vi "PH_Beckhoff_PP_Control.write Mercury to PSDB.vi"(0 "i ref in":refnum<vi>, 5 "error IO":errorcluster) -> (14 "i ref out":refnum<vi>, 19 "error out":errorcluster)   [LabVIEW 2014, in "PH_Beckhoff_PP_Control.lvlib"]
doc: "This VI writes the mercury data to the PHELIX shot data base."
uses:
  PH_Beckhoff_PP_Control.lvlib
  PH_Basics/PH_StatusHandler/PH_StatusHandler.Status.ctl
  PH_Basics/PH_PSDBWriter/PH_PSDBWriter.Data Status.ctl
  PH_Beckhoff/PH_Beckhoff.lvlib
  CS_Core/CSSystem/CSSystemLib/CSSystemLib.lvlib
  PH_Basics/PH_PSDBWriter/PH_PSDBWriter.lvlib
  PH_Basics/PH_Common/PH_Common.lvlib
  PH_Basics/PH_StatusHandler/PH_StatusHandler.lvlib
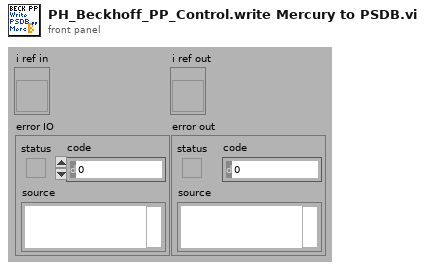
[diagram p1: front panel]
types:
  T1 = typedef "PH_Beckhoff.lvlib/PH_Beckhoff.i attribute.ctl" = cluster{"GUI Refs":T2, "operation?":bool, "Default Prdc Interval":i32, "Connection":T3, "AMS Net ID":T4, "Klemmencluster: # of":T5, "Values":T6, "IP":string, "Description":string, "configured?":bool, "Change Manager":cluster{"Detemination wanted?":bool, "Values changed at":cluster{"Sonderklemmen Inputs":i32[], "Analog Inputs":i32[], "Analog Outputs":i32[], "Digital Inputs":i32[], "Digital Outputs":i32[]}}, "Difference to handle an analog input as change":u32}
  T2 = typedef "PH_Beckhoff.lvlib/PH_Beckhoff.GUI Refs.ctl" = cluster{"ADS Error":refnum<vi>, "Values":refnum<vi>, "configured?":refnum<vi>, "Connection":refnum<vi>, "IP":refnum<vi>, "Prdc Int [ms]":refnum<vi>}
  T3 = typedef "PH_Beckhoff.lvlib/PH_Beckhoff.Connectivity.ctl" = cluster{"DLL?":bool, "Port?":bool, "Client?":bool, "Ping?":bool, "unsuccessful Pings":u32}
  T4 = typedef "Beckhoff - Driver np.lvlib/Beckhoff Access.ctl" = cluster{"DLL path":path, "AMS Net ID":cluster{"1st # of IP":u8, "2nd # of IP":u8, "3rd # of IP":u8, "4th # of IP":u8, "In Port":u8, "Out Port":u8}}
  T5 = typedef "Beckhoff - Driver np.lvlib/Klemmendeclarer.ctl" = cluster{"Offset due to Sonderklemms":u32, "analog Inputs":u32, "analog Outputs":u32, "digital Input Bits":u32, "digital Output Bits":u32}
  T6 = typedef "PH_Beckhoff.lvlib/PH_Beckhoff.Values.ctl" = cluster{"Sonderklemmen Inputs":T7, "Analog Inputs":T8, "Analog Outputs":T10, "Digital Inputs":T11, "Digital Outputs":T12}
  T7 = typedef "PH_Beckhoff.lvlib/PH_Beckhoff.Sonderklemmen Inputs.ctl" = cluster{"Total Length":u32, "Name":string, "Value":u64, "Quality":bool, "Service ID":i32, "Offset":u32, "Length":u32}[]
  T8 = typedef "PH_Beckhoff.lvlib/PH_Beckhoff.Analog Inputs.ctl" = cluster{"Name":string, "Value":u32, "Quality":bool, "Service ID":i32, "Sca Type":T9}[]
  T9 = typedef "PH_Beckhoff.lvlib/PH_Beckhoff.Scaling Type.ctl" = enum16{"none", "0 ... 15 Bit -> 0 ... 5", "0 ... 15 Bit -> 0 ... 10", "0 ... 15 Bit -> 0 ... 25", "0 ... 15 Bit -> 4 ... 20", "0 ... 15 Bit -> 0 ... 1", "0 ... 15 Bit -> 0 ... 20000", "0 ... 15 Bit -> 0 ... 24000"}
  T10 = typedef "PH_Beckhoff.lvlib/PH_Beckhoff.Analog Outputs.ctl" = cluster{"Name":string, "Value":u32, "Quality":bool, "Wanted Value":u32, "Service ID":i32, "Sca Type":T9}[]
  T11 = typedef "PH_Beckhoff.lvlib/PH_Beckhoff.Digital Inputs.ctl" = cluster{"Name":string, "Value":bool, "Quality":bool, "Service ID":i32, "inverted?":bool}[]
  T12 = typedef "PH_Beckhoff.lvlib/PH_Beckhoff.Digital Outputs.ctl" = cluster{"Name":string, "Value":bool, "Quality":bool, "Wanted Value":bool, "Service ID":i32, "inverted?":bool}[]
  T13 = typedef "PH_Beckhoff_PP_Control.lvlib/PH_Beckhoff_PP_Control.i attribute.ctl" = cluster{"PP Conductivity Control":cluster{"PSDB":cluster{"Status Service ID":i32, "Instance ID":i32, "Data Status":T14, "Ref Status":refnum<vi>, "Error Code":i32}, "Status":cluster{"GUI Ref":refnum<vi>, "Status Service ID":i32, "Status":T15}, "DIs":cluster{"Device on":cluster{"GUI Ref":refnum<vi>, "# in Data":i32}, "Conductivity ok":cluster{"GUI Ref":refnum<vi>, "# in Data":i32}, "Temperature ok":cluster{"GUI Ref":refnum<vi>, "# in Data":i32}, "Alarm":cluster{"GUI Ref":refnum<vi>, "# in Data":i32}}, "PSDB Thread":cluster{"Ref":refnum<vi>, "Q-Ref":refnum<queue>}}, "PP Mercury Control":cluster{"PSDB":cluster{"Status Service ID":i32, "Instance ID":i32, "Data Status":T14, "Ref Status":refnum<vi>, "Error Code":i32}, "Status":cluster{"GUI Ref":refnum<vi>, "Status Service ID":i32, "Status":T15}, "on since:":cluster{"GUI Ref":refnum<vi>, "Service ID":i32, "Time":string}, "DIs":cluster{"Device on":cluster{"GUI Ref":refnum<vi>, "# in Data":i32}, "Alarm":cluster{"GUI Ref":refnum<vi>, "# in Data":i32}}, "AIs":cluster{"Concentration":cluster{"GUI Ref":refnum<vi>, "# in Data":i32}}, "PSDB Thread":cluster{"Ref":refnum<vi>, "Q-Ref":refnum<queue>}}, "PSDB":cluster{"Shot #":i32, "Subsystem":T16}, "PSDB Credentials":T17}
  T14 = typedef "PH_PSDBWriter.lvlib/PH_PSDBWriter.Data Status.ctl" = i16
  T15 = typedef "PH_StatusHandler.lvlib/PH_StatusHandler.Status.ctl" = i16
  T16 = typedef "PH_PSDBWriter.lvlib/PH_PSDBWriter.PHELIX-Subsystems.ctl" = i32
  T17 = typedef "PH_Common.lvlib/PH_Connection.PSDB Credentials.ctl" = cluster{"PW":string, "ID":string, "DS":string}
  T18 = typedef "PH_PSDBWriter.lvlib/PH_PSDBWriter.Numeric dataset.ctl" = cluster{"name":string, "data":dbl, "unit":string}
  T19 = typedef "PH_PSDBWriter.lvlib/PH_PSDBWriter.String dataset.ctl" = cluster{"name":string, "data":string, "unit":string}
  T20 = typedef "PH_PSDBWriter.lvlib/PH_PSDBWriter.PSDB Dataset.ctl" = cluster{"Version":i32, "2D data Input":T21[], "Boolean Input":T23[], "Image Input":T24[], "Numeric Input":T18[], "String Input":T19[]}
  T21 = typedef "PH_PSDBWriter.lvlib/PH_PSDBWriter.2D dataset.ctl" = cluster{"name":string, "data":dbl[][], "axis description":T22}
  T22 = typedef "PSDB.lvlib/PSDB_AxisDescription.ctl" = cluster{"x axis label":string, "y axis label":string, "x axis unit":string, "y axis unit":string}
  T23 = typedef "PH_PSDBWriter.lvlib/PH_PSDBWriter.Boolean dataset.ctl" = cluster{"name":string, "data":bool, "unit":string}
  T24 = typedef "PH_PSDBWriter.lvlib/PH_PSDBWriter.Image dataset.ctl" = cluster{"name":string, "data":T25, "unit":string}
  T25 = typedef "IMAQ Image.ctl" = refnum<image>
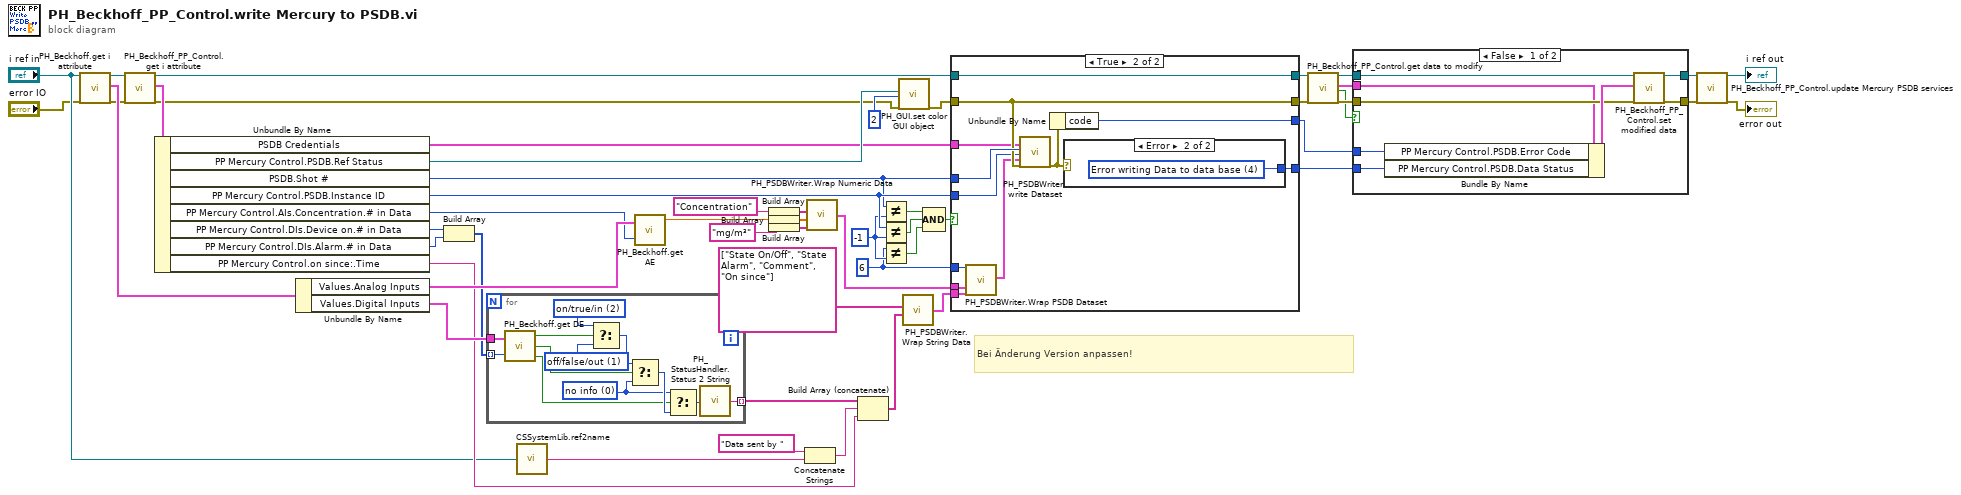
[diagram p0: block diagram]
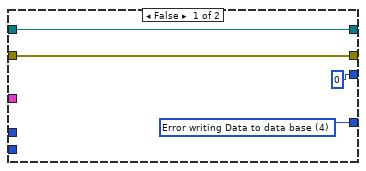
[diagram p3: hidden frame]
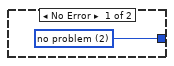
[diagram p4: hidden frame]
diagram:
  w41 = 6 ("Version")
  w47 = -1 ("y")
  # "Bei Änderung Version anpassen!"
  n1 = call "PH_Beckhoff.get i attribute.vi"("i ref in"="i ref in", "error in (no error)"="error IO") -> ("i ref out"=w40:refnum<vi>, "i attribute"=w39:T1, "error out"=w19:errorcluster)  [unwired: 15 in]
  n2 = call "PH_Beckhoff_PP_Control.get i attribute.vi"("i ref in"=w40, "error in (no error)"=w19) -> ("i ref out"=w20:refnum<vi>, "i attribute"=w16:T13, "error out"=w13:errorcluster)  [unwired: 15 in]
  n3 = Unbundle By Name(w16) -> ("PSDB Credentials"=w1:T17, "PP Mercury Control.PSDB.Ref Status"=w14:refnum<vi>, "PSDB.Shot #"=w50:i32, "PP Mercury Control.PSDB.Instance ID"=w51:i32, "PP Mercury Control.AIs.Concentration.# in Data"=w37:i32, "PP Mercury Control.DIs.Device on.# in Data"=w35:i32, "PP Mercury Control.DIs.Alarm.# in Data"=w34:i32, "PP Mercury Control.on since:.Time"=w28:string)
  n4 = Unbundle By Name(w39) -> ("Values.Analog Inputs"=w38:T8, "Values.Digital Inputs"=w36:T11)
  n5 = Build Array(w35, w34) -> (w33:i32[])
  n6 = for {
    tunnel: [w59] -> w32 mode=indexing
    tunnel: w36 -> [w55]
    tunnel: w33 -> [w54] mode=indexing
    w61 = T15 1 items=["no info", "off/false/out", "on/true/in", "Failure", "Alarm", "Status 1", "Status 2", "Status 3"] ("State Temp not 2 low")
    w62 = T15 2 items=["no info", "off/false/out", "on/true/in", "Failure", "Alarm", "Status 1", "Status 2", "Status 3"] ("State Temp not 2 low")
    w64 = T15 0 items=["no info", "off/false/out", "on/true/in", "Failure", "Alarm", "Status 1", "Status 2", "Status 3"] ("State Temp not 2 low")
    n7 = call "PH_Beckhoff.get DE.vi"("Digital Values"=w55, "index of element"=w54) -> ("Value"=w58:bool, "Quality"=w57:bool, "Tag not found"=w56:bool)
    n8 = Select(t=w62, s=w58, f=w61) -> (s? t:f=w63:T15)
    n9 = Select(t=w63, s=w57, f=w64) -> (s? t:f=w65:T15)
    n10 = Select(t=w64, s=w56, f=w65) -> (s? t:f=w60:T15)
    n11 = call "PH_StatusHandler.Status 2 String.vi"("Status"=w60) -> ("Status as string"=w59:string)
  }
  n12 = call "CSSystemLib.ref2name.vi"("obj refnum"="i ref in") -> ("name"=w30:string)
  n13 = call "PH_Beckhoff.get AE.vi"("Analog Inputs"=w38, "index of element"=w37) -> ("DIM value"=w9:dbl)  [unwired: 2 out]
  n14 = Build Array("Concentration" ("name")) -> (w6:string[])
  n15 = Build Array(w9) -> (w8:dbl[])
  n16 = Build Array("mg/m³" ("unit")) -> (w4:string[])
  n17 = Concatenate Strings("Data sent by " ("string"), w30) -> (w29:string)
  n18 = call "PH_PSDBWriter.Wrap Numeric Data.vi"("Unit Array"=w4, "Data Array"=w8, "Name Array"=w6) -> ("PSDB Numeric Data Array"=w3:T18[])  [unwired: 1 in]
  n19 = Build Array (concatenate)(w32, w29, w28) -> (w10:string[])
  n20 = Not Equal?(x=w50, y=w47) -> (x != y?=w46:bool)
  n21 = Not Equal?(x=w51, y=w47) -> (x != y?=w45:bool)
  n22 = Not Equal?(x=w41, y=w47) -> (x != y?=w44:bool)
  n23 = call "PH_GUI.set color GUI object.vi"("GUI object Ref"=w14, "State"=2, "error in (no error)"=w13) -> ("error out"=w12:errorcluster)  [unwired: 16 in]
  n24 = call "PH_PSDBWriter.Wrap String Data.vi"("Data Array"=w10, "Name Array"=string[] ["State On/Off", "State Alarm", "Comment", "On since"]) -> ("PSDB String Data Array"=w2:T19[])  [unwired: 2 in]
  n25 = Compound Arithmetic op=AND(w46, w45, w44) -> (w43:bool)
  n26 = case shown="True" w43 {
    tunnel: w12 -> [w67 w77]
    tunnel: w51 -> [_ w74]
    tunnel: w41 -> [_ w71]
    tunnel: [w69 w81] -> w48
    tunnel: w20 -> [w68 w80]
    tunnel: [w68 w80] -> w26
    tunnel: [w67 w77] -> w24
    tunnel: w50 -> [_ w78]
    tunnel: [0 ("code") w79] -> w42
    tunnel: w3 -> [_ w73]
    tunnel: w2 -> [_ w72]
    tunnel: w1 -> [_ w70]
    frame False {
      w69 = T14 4 items=["no info", "no Data collection", "no problem", "Error getting the instance ID", "Error writing Data to data base", "Error concerning the subsystem"] ("Data Status")
    }
    frame True {
      n27 = call "PH_PSDBWriter.Wrap PSDB Dataset.vi"("Version"=w71, "Numeric Input"=w73, "String Input"=w72) -> ("PSDB Dataset"=w75:T20)  [unwired: 16 in]
      n28 = call "PH_PSDBWriter.write Dataset.vi"("PSDB Credentials"=w70, "Shot #"=w78, "Instance ID"=w74, "Data to write to PSDB"=w75, "error in (no error)"=w77) -> ("error out"=w76:errorcluster)  [unwired: 14 in]
      n29 = Unbundle By Name(w76) -> ("code"=w79:i32)
      n30 = case shown="Error" w76 {
        tunnel: [w82 w83] -> w81
        frame No Error {
          w82 = T14 2 items=["no info", "no Data collection", "no problem", "Error getting the instance ID", "Error writing Data to data base", "Error concerning the subsystem"] ("Data Status")
        }
        frame Error {
          w83 = T14 4 items=["no info", "no Data collection", "no problem", "Error getting the instance ID", "Error writing Data to data base", "Error concerning the subsystem"] ("Data Status")
        }
      }
    }
  }
  n31 = call "PH_Beckhoff_PP_Control.get data to modify.vi"("i ref in"=w26, "error in (no error)"=w24) -> ("i ref out"=w27:refnum<vi>, "i attribute"=w23:T13, "timed out"=w22:bool, "error out"=w25:errorcluster)  [unwired: 14 in]
  n32 = case shown="False" w22 {
    tunnel: [w91 w93] -> w21
    tunnel: [w90 w92] -> w49
    tunnel: w48 -> [w89 _]
    tunnel: w42 -> [w87 _]
    tunnel: w27 -> [w86 w93]
    tunnel: w25 -> [w85 w92]
    tunnel: w23 -> [w84 _]
    frame False {
      n33 = Bundle By Name(cluster=w84, "PP Mercury Control.PSDB.Error Code"=w87, "PP Mercury Control.PSDB.Data Status"=w89) -> (w88:T13)
      n34 = call "PH_Beckhoff_PP_Control.set modified data.vi"("i ref in"=w86, "i attribute"=w88, "error in (no error)"=w85) -> ("i ref out"=w91:refnum<vi>, "error out"=w90:errorcluster)  [unwired: 15 in]
    }
    frame True {
    }
  }
  n35 = call "PH_Beckhoff_PP_Control.update Mercury PSDB services.vi"("i ref in"=w21, "error in"=w49) -> ("i ref out"=→"i ref out":refnum<vi>, "error out"=→"error out":errorcluster)  [unwired: 16 in]
